vi "Prototype.vi"(8 "error in (no error)":errorcluster, 10 "Abstract Prototyper in":refnum<class "Abstract Icon Prototyper.lvclass">, 11 "Scripter in":refnum<class "Message Scripter.lvclass">) -> (0 "error out":errorcluster, 2 "Abstract Prototyper out":refnum<class "Abstract Icon Prototyper.lvclass">, 3 "Scripter out":refnum<class "Message Scripter.lvclass">)   [LabVIEW 2020, in "Message Maker.lvlib" / "Abstract Icon Prototyper.lvclass"]
uses:
  Abstract Icon Prototyper.lvclass
  <vilib>/picture/picture.llb/imagedata.ctl
  Message Scripter/Message Scripter.lvclass
  Message Maker.lvlib
  <vilib>/Utility/miscctls.llb/LVPoint32TypeDef.ctl
  <vilib>/LabVIEW Icon API/API_User Layer Data.ctl
  <vilib>/LabVIEW Icon API/LabVIEW Icon API.lvlib
  _support/Localized Strings.vi
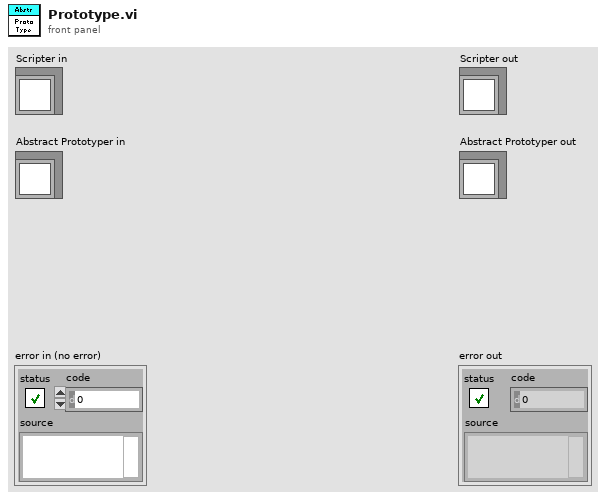
[diagram p1: front panel]
types:
  T1 = typedef "LabVIEW Icon API.lvlib/API_User Layer Data.ctl" = cluster{"Layer name":string, "Origin":T2, "Icon image data":T3}
  T2 = typedef "LVPoint32TypeDef.ctl" = cluster{"Horizontal":i32, "Vertical":i32}
  T3 = typedef "imagedata.ctl" = cluster{"image type":i32, "image depth":i32, "image":u8[], "mask":u8[], "colors":u32[], "Rectangle":cluster{"left":i16, "top":i16, "right":i16, "bottom":i16}}
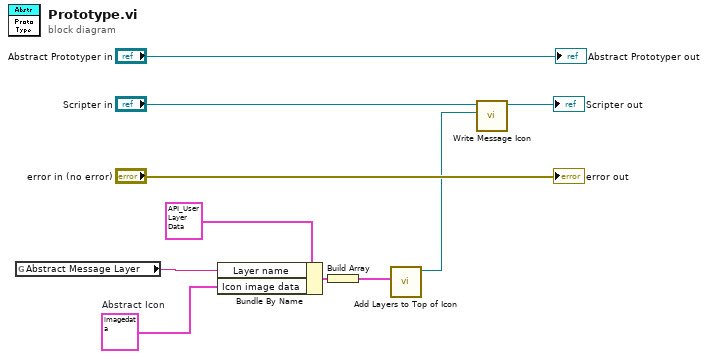
[diagram p0: block diagram]
diagram:
  w5 = T3 {"image type"=0, "image depth"=24, "image"=array[3072 elements], "mask"=[255, 255, 255, 255, 128, 0, 0, 1, 128, 63, 252, 1, 128, 32, 4, 1, 128, 47, 244, 1, 128, 47, 244, 1, 128, 47, 244, 1, 128, 47, 244, 1, 128, 32, 4, 1, 128, 63, 252, 1, 128, 0, 0, 1, 255, 255, 255, 255, 128, 0, 0, 1, 128, 0, 0, 1, 128, 0, 0, 1, 128, 1, 224, 1, 128, 7, 248, 1, 128, 31, 254, 1, 128, 31, 254, 1, 128, 31, 254, 1, 128, 31, 254, 1, 128, 31, 254, 1, 128, 31, 254, 1, 128, 31, 254, 1, 128, 31, 254, 1, 128, 31, 254, 1, 128, 31, 254, 1, 128, 7, 248, 1, 128, 1, 224, 1, 128, 0, 0, 1, 128, 0, 0, 1, 255, 255, 255, 255], "colors"=[], "Rectangle"={"left"=0, "top"=0, "right"=32, "bottom"=32}}  # Abstract Icon
  n1 = global read "Localized Strings.vi" "Abstract Message Layer"() -> (w1:string)
  n2 = Bundle By Name(cluster=T1 {"Layer name"="", "Origin"={"Horizontal"=0, "Vertical"=0}, "Icon image data"={"image type"=0, "image depth"=0, "image"=[], "mask"=[], "colors"=[], "Rectangle"={"left"=0, "top"=0, "right"=0, "bottom"=0}}} ("User layer"), "Layer name"=w1, "Icon image data"=w5) -> (w4:T1)
  n3 = Build Array(w4) -> (w3:T1[])
  n4 = call "Add Layers to Top of Icon.vi"("User layers"=w3) -> ("Icon.lvclass out"=w2:refnum<class "Icon.lvclass">)  [unwired: 10 in]
  n5 = call-dynamic "Write Message Icon.vi"("Message Icon"=w2, "Message Scripter in"="Scripter in") -> ("Message Scripter out"=→"Scripter out":refnum<class "Message Scripter.lvclass">)  [unwired: 9 in]
  "error out" <- "error in (no error)"
  "Abstract Prototyper out" <- "Abstract Prototyper in"
